vi "practice08_servo_control.vi"() -> ()   [LabVIEW 2025]
uses:
  <vilib>/Instr/_visa.llb/VISA Configure Serial Port (Instr).vi
panel:
  out "Grados recibidos":i32(knob) scale=0.0..180.0
  in  "Selección de grados":u8(knob) scale=0.0..180.0
  in  "stop":bool
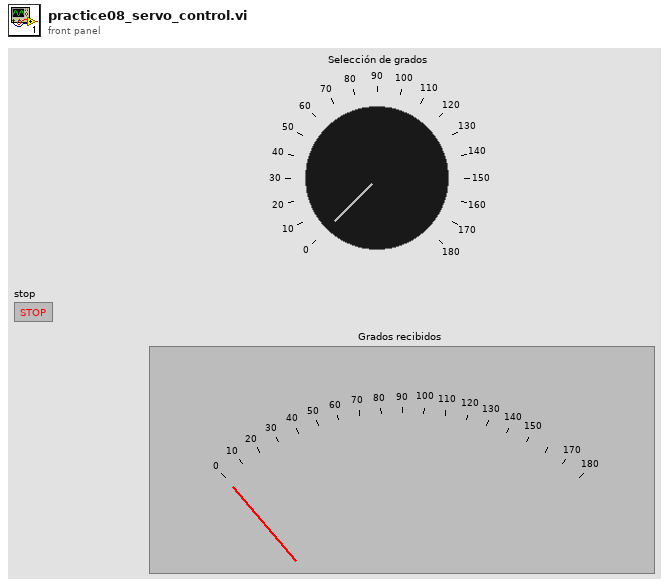
[diagram p1: front panel]
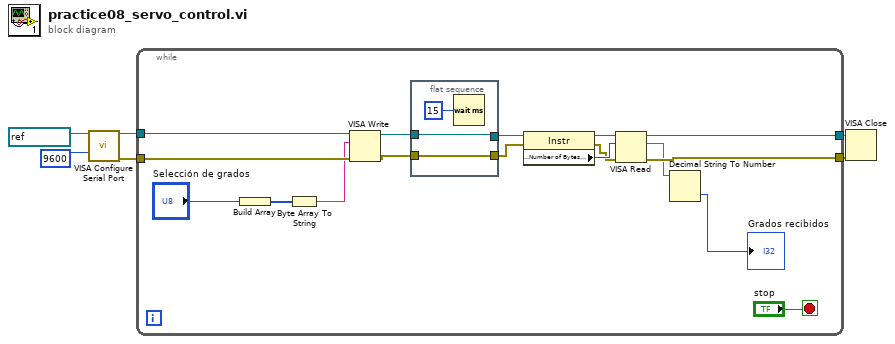
[diagram p0: block diagram]
diagram:
  n1 = call-poly "VISA Configure Serial Port"("VISA resource name"=refnum<visa-resource-name> "COM3", "parity (0:none)"=9600) -> ("VISA resource name out"=w3:refnum<visa-resource-name>, "error out"=w4:errorcluster)  [unwired: 12 in]
  n2 = while {
    tunnel: w4 -> [w22]
    tunnel: w3 -> [w21]
    tunnel: [w10] -> w2
    tunnel: [w9] -> w1
    stop <- "stop" stop-if-true
    n3 = Build Array("Selección de grados") -> (w19:u8[])
    n4 = Byte Array To String(unsigned byte array=w19) -> (string=w20:string)
    n5 = VISA Write(VISA resource name=w21, write buffer=w20, error in (no error)=w22) -> (VISA resource name out=w16:refnum<visa-resource-name>, error out=w17:errorcluster)  [unwired: 1 out]
    n6 = flat-sequence {
      tunnel: [w25] -> w18
      tunnel: w17 -> [w25]
      tunnel: [w24] -> w15
      tunnel: w16 -> [w24]
      frame #0 {
        n7 = Wait (ms)(milliseconds to wait=u32 15) -> ()  [unwired: 1 out]
      }
    }
    n8 = property class="Instr"(reference=w15, error in=w18) -> (reference out=w13:refnum<visa-resource-name>, error out=w11:errorcluster, "Serial Settings:Number of Bytes at Serial Port"=w12:u32)
    n9 = VISA Read(VISA resource name=w13, byte count=w12, error in (no error)=w11) -> (VISA resource name out=w9:refnum<visa-resource-name>, read buffer=w8:string, error out=w10:errorcluster)  [unwired: 1 out]
    n10 = Decimal String To Number(string=w8) -> (number=→"Grados recibidos":i32)  [unwired: 2 in, 1 out]
  }
  n11 = VISA Close(VISA resource name=w1, error in (no error)=w2) -> ()  [unwired: 1 out]
